vi "ISX3_Cmd_SetSetupStartCalibration.vi"() -> (0 "set Setup Start Calibration Cmd":u8[](array[numeric]))   [LabVIEW 2012, in "Sciospec ISX3 Impedance Analyzer.lvlib"]
uses:
  Sciospec ISX3 Impedance Analyzer.lvlib
panel:
  # "This VI generates the command to initate the calibration sequence for a configurated setup.\nAny previous calibration data for the configured setup is cleared."
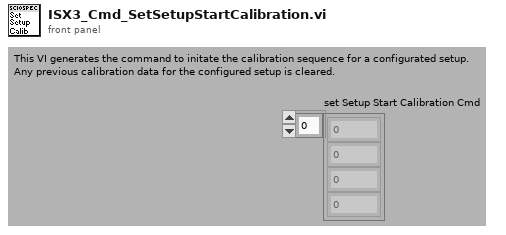
[diagram p1: front panel]
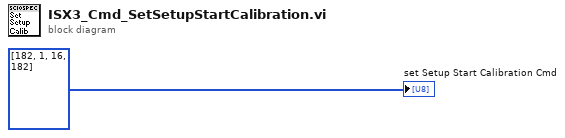
[diagram p0: block diagram]
diagram:
  "set Setup Start Calibration Cmd" <- u8[] [182, 1, 16, 182]
